vi "Add Test Registration.vi"(8 "error in (no error)":errorcluster, 10 "Test Registration":T1, 11 "Test Event Storage in":refnum<class "Test Event Storage.lvclass">) -> (0 "error out":errorcluster, 2 "updated?":bool, 3 "Test Event Storage out":refnum<class "Test Event Storage.lvclass">)   [LabVIEW 2009, in "Caraya.lvlib" / "Test Event Storage.lvclass"]
uses:
  Test Event Storage.lvclass
  Basic Test Manager/Test Registration Data.ctl
  Test Node.ctl
  Test Event Storage.lvclass/Test Event Storage.ctl
  Basic Test Manager/Basic Test Manager.lvclass
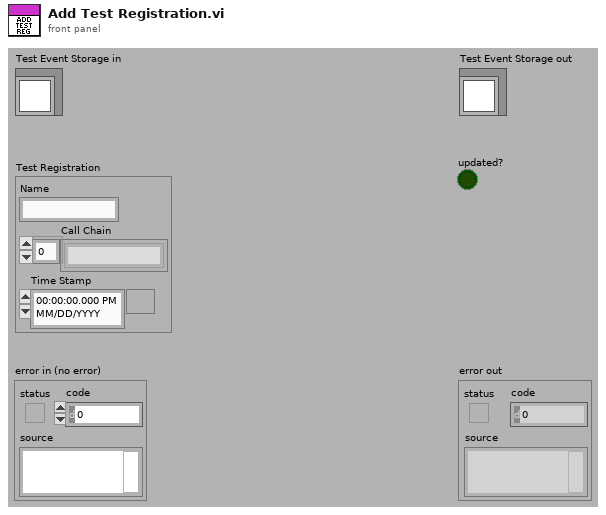
[diagram p1: front panel]
types:
  T1 = typedef "Caraya.lvlib/Basic Test Manager.lvclass/Test Registration Data.ctl" = cluster{"Name":string, "Call Chain":string[], "Time Stamp":timestamp}
  T2 = typedef "Caraya.lvlib/Test Event Storage.lvclass/Test Node.ctl" = cluster{"Test Registration":T1, "Defined":bool, "Passed":bool}
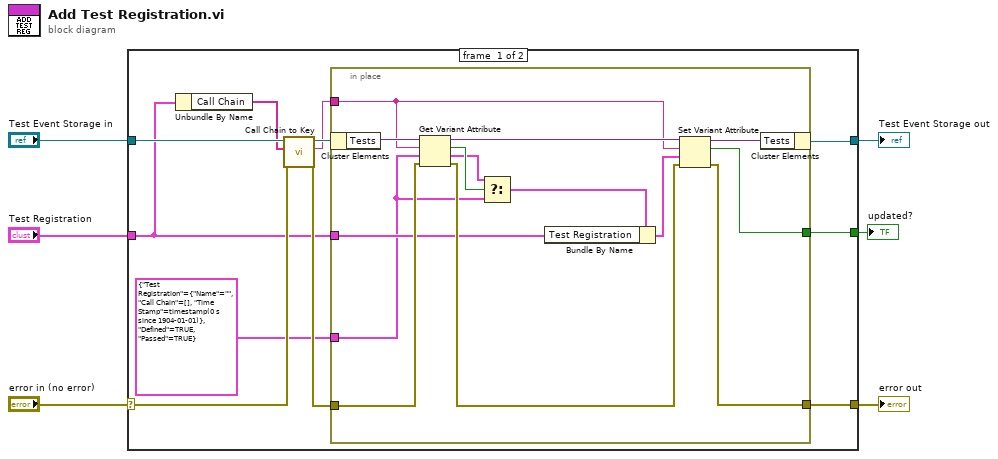
[diagram p0: block diagram]
diagram:
  n1 = case shown="No Error" "error in (no error)" {
    selector: "error in (no error)" -> [w15 w33]
    tunnel: [w11 w33] -> w5
    tunnel: [w10 w32] -> w3
    tunnel: "Test Event Storage in" -> [w17 w32]
    tunnel: "Test Registration" -> [w9 _]
    tunnel: [w8 _] -> w1
    frame #0 {
      n2 = Unbundle By Name(w9) -> ("Call Chain"=w13:string[])
      n3 = call "Call Chain to Key.vi"("error in (no error)"=w15, "Call Chain"=w13, "Test Event Storage in"=w17) -> ("error out"=w14:errorcluster, "Key"=w12:string, "Test Event Storage out"=w16:refnum<class "Test Event Storage.lvclass">)  [unwired: 6 in]
      n4 = in-place {
        in-place-border: w14 -> [w26]
        in-place-border: w12 -> [w24]
        in-place-border: w9 -> [w23]
        in-place-border: [w30] -> w11
        in-place-border: [w29] -> w8
        in-place-border: T2 {"Test Registration"={"Name"="", "Call Chain"=[], "Time Stamp"=timestamp(0 s since 1904-01-01)}, "Defined"=TRUE, "Passed"=TRUE} ("Test Node") -> [w19]
        n5 = in-place-cluster #1(w16) -> ("Tests"=w28:variant)
        n6 = Get Variant Attribute(Variant=w28, name=w24, default value (empty Variant)=w19, error in=w26) -> (duplicate Variant=w27:variant, found=w21:bool, value=w20:T2, error out=w25:errorcluster)
        n7 = Select(t=w20, s=w21, f=w19) -> (s? t:f=w18:T2)
        n8 = Bundle By Name(cluster=w18, "Test Registration"=w23) -> (w22:T2)
        n9 = Set Variant Attribute(Variant=w27, name=w24, value=w22, error in=w25) -> (Variant out=w31:variant, replaced=w29:bool, error out=w30:errorcluster)
        n10 = in-place-cluster #1("Tests"=w31) -> (w10:refnum<class "Test Event Storage.lvclass">)
      }
    }
    frame #1 {
    }
  }
  "error out" <- w5
  "Test Event Storage out" <- w3
  "updated?" <- w1
